vi "ex7_2.vi"() -> ()   [LabVIEW 2022 SP3]
panel:
  in  "?":bool
  in  "Reset Timer":bool
  out "Elapsed Time [ms]":dbl format="%#_4g"
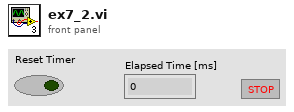
[diagram p1: front panel]
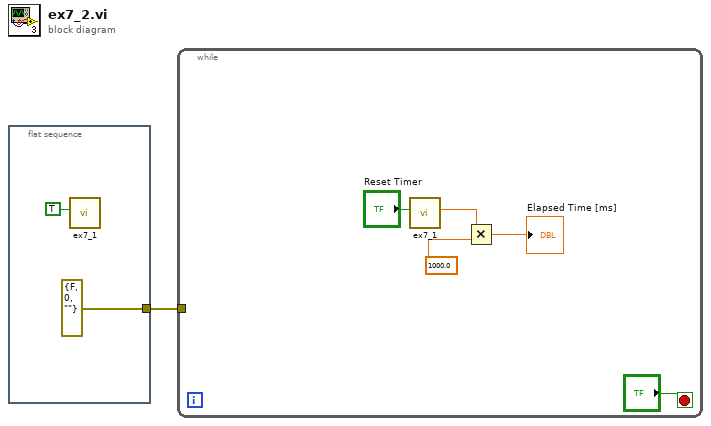
[diagram p0: block diagram]
diagram:
  n1 = flat-sequence {
    tunnel: [errorcluster {"status"=FALSE, "code"=0, "source"=""} ("error constant")] -> w1
    frame #0 {
      n2 = call "ex7_1.vi"("Reset Timer"=TRUE ("Reset")) -> ()  [unwired: 10 in, 1 out]
    }
  }
  n3 = while {
    tunnel: w1 -> [_]
    stop <- "?" stop-if-true
    n4 = call "ex7_1.vi"("Reset Timer"="Reset Timer") -> ("Elapsed Time [ms]"=w5:dbl)  [unwired: 10 in]
    n5 = Multiply(x=w5, y=1000.0) -> (x*y=→"Elapsed Time [ms]":dbl)
  }
